vi "MovingZ.vi"   [LabVIEW 2016]
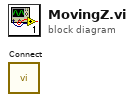
[diagram p0: block diagram]
diagram:
  n1 = call "Connect.vi"() -> ()  [unwired: 10 in, 2 out]
